vi "Drop Message Core.vi"(11 "CyclicMessage in":refnum<class "MessageCycle.lvclass">) -> ()   [LabVIEW 2020, in "MessageCycle.lvclass"]
doc: "(<B>Filename</B>: Actor Framework.lvlib:Message.lvclass:Drop Message Core.vi)\n\nDefines what a message does if it is in the message queue when the queue is released. At this point, the actor has shut down, so it will never process the message.\n\nBy default, this method does nothing. A child class may override it to define behavior. National Instruments provides the Reply Msg class to override this method. This class releases its internal queue, which causes any caller of the Send Message and Wait For Response method to stop waiting and return an error."
uses:
  <vilib>/gpm_packages/@cs/actor-framework-messages/Source/MessageCycle/MessageCycle.lvclass
  <vilib>/gpm_packages/@cs/actor-framework-messages/Source/MessageCycle/MessageCycle.lvclass/MessageCycle.ctl
  <vilib>/ActorFramework/Message/Message.lvclass
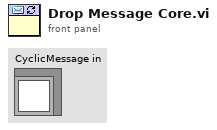
[diagram p1: front panel]
types:
  T1 = typedef "MessageCycle.lvclass/Message Cycle Notifications.ctl" = enum16{"Process Final Copy and Stop", "Stop Immediately", "Substitute Last Message and Stop"}
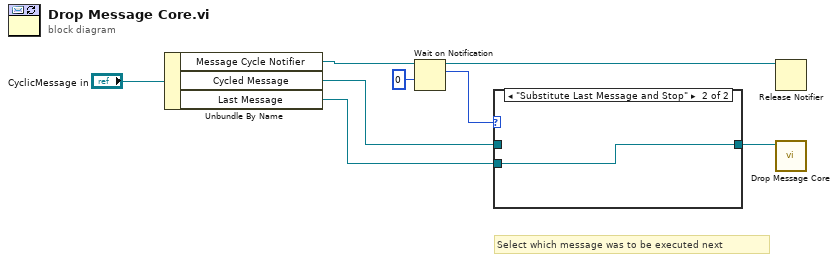
[diagram p0: block diagram]
diagram:
  # "Select which message was to be executed next"
  n1 = Unbundle By Name("CyclicMessage in") -> ("Message Cycle Notifier"=w7:refnum<notifier>, "Cycled Message"=w6:refnum<class "Message.lvclass">, "Last Message"=w2:refnum<class "Message.lvclass">)
  n2 = Wait on Notification(notifier=w7, timeout in ms (-1)=0) -> (notifier out=w5:refnum<notifier>, notification=w3:T1)  [unwired: 2 in, 2 out]
  n3 = case shown="\"Substitute Last Message and Stop\"" w3 {
    tunnel: w6 -> [w9 _]
    tunnel: w2 -> [_ w10]
    tunnel: [w9 w10] -> w1
    frame Default {
    }
    frame "Substitute Last Message and Stop" {
    }
  }
  n4 = Release Notifier(notifier=w5) -> ()  [unwired: 2 in, 3 out]
  n5 = call-dynamic "Drop Message Core.vi"("Message in"=w1) -> ()  [unwired: 11 in]
